vi "measuretime.vi"() -> ()   [LabVIEW 2021]
panel:
  out "total time":u32
  out "F(n)":i32
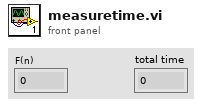
[diagram p1: front panel]
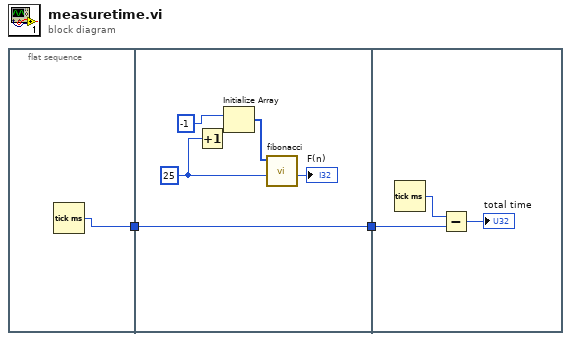
[diagram p0: block diagram]
diagram:
  n1 = flat-sequence {
    tunnel: [w3] -> w2
    tunnel: w2 -> [w8]
    tunnel: [w8] -> w1
    tunnel: w1 -> [w11]
    frame #0 {
      n2 = Tick Count (ms)() -> (millisecond timer value=w3:u32)
    }
    frame #1 {
      w7 = u8 25 ("n")
      n3 = Increment(x=w7) -> (x+1=w4:u8)
      n4 = Initialize Array(-1, w4) -> (w5:i32[])
      n5 = call "fibonacci.vi"("n"=w7, "cache in"=w5) -> ("F(n)"=→"F(n)":i32)  [unwired: 8 in, 1 out]
    }
    frame #2 {
      n6 = Tick Count (ms)() -> (millisecond timer value=w12:u32)
      n7 = Subtract(x=w12, y=w11) -> (x-y=→"total time":u32)
    }
  }
